vi "PidHmiTwoWordToFloat.vi"(10 "register 2":u16, 11 "register 1":u16) -> (3 "number":sgl)   [LabVIEW 2018, in "Pid.lvlib"]
uses:
  Pid.lvlib
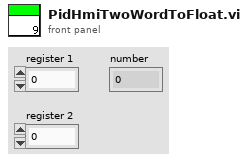
[diagram p1: front panel]
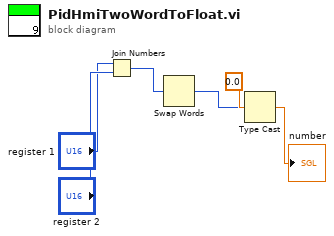
[diagram p0: block diagram]
diagram:
  n1 = Join Numbers(hi="register 1", lo="register 2") -> ((hi.lo)=w1:u32)
  n2 = Swap Words(1:w1) -> (0:w4:u32)
  n3 = Type Cast(type=sgl 0.0 ("number"), x=w4) -> (*(type *) &x=→"number":sgl)
